vi "Limit Test.vi"(7 "CallingVI":refnum<vi>, 8 "error in":errorcluster, 9 "Previous":dbl, 10 "Setpoint in":dbl, 11 "Limits in":cluster{"Maximum":dbl, "Minimum":dbl}) -> (0 "error out":errorcluster, 2 "Setpoint out":dbl, 3 "Limits out":cluster{"Maximum":dbl, "Minimum":dbl})   [LabVIEW 2023, in "Instruments.lvlib" / "Instruments.lvclass"]
doc: "This routine tests limits provided by the caller routine and generates a warning if the value is out of range."
uses:
  Library/Instruments.lvclass
  <vilib>/ErrorRing/Error Ring.xnode
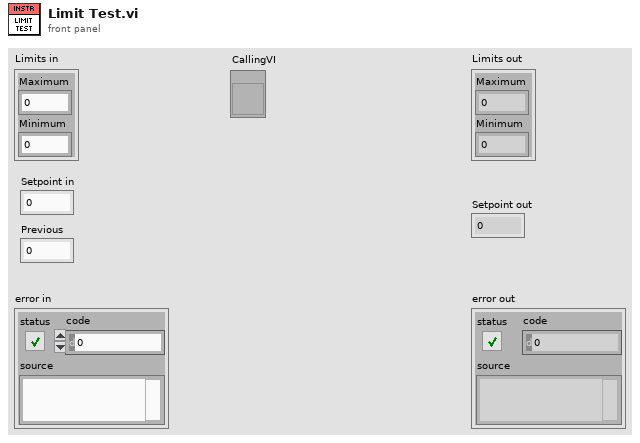
[diagram p1: front panel]
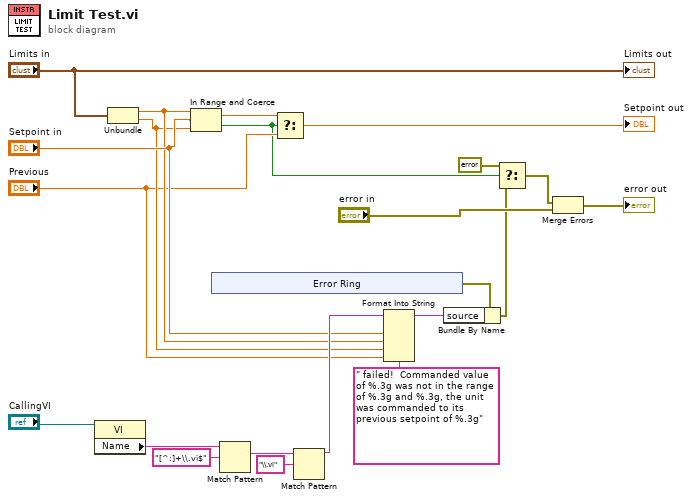
[diagram p0: block diagram]
diagram:
  n1 = property class="VI"(reference="CallingVI") -> ("Name"=w15:string)  [unwired: 1 in, 2 out]
  n2 = Unbundle("Limits in") -> ("Maximum"=w11:dbl, "Minimum"=w10:dbl)
  n3 = In Range and Coerce(upper limit=w11, x="Setpoint in", lower limit=w10) -> (coerced(x)=w21:dbl, In Range?=w6:bool)
  n4 = xnode "Error Ring"() -> ("error out"=w8:errorcluster)
  n5 = Match Pattern(string=w15, regular expression="[^:]+\\.vi$") -> (match substring=w17:string)  [unwired: 1 in, 3 out]
  n6 = Select(t=w21, s=w6, f="Previous") -> (s? t:f=→"Setpoint out":dbl)
  n7 = Match Pattern(string=w17, regular expression="\\.vi") -> (before substring=w13:string)  [unwired: 1 in, 3 out]
  n8 = Format Into String(format string=" failed!  Commanded value of %.3g was not in the range of %.3g and %.3g, the unit was commanded to its previous setpoint of %.3g", initial string=w13, "Setpoint in", w11, w10, "Previous") -> (resulting string=w7:string)  [unwired: 1 in, 1 out]
  n9 = Bundle By Name(cluster=w8, "source"=w7) -> (w2:errorcluster)
  n10 = Select(t=errorcluster {"status"=FALSE, "code"=0, "source"=""}, s=w6, f=w2) -> (s? t:f=w5:errorcluster)
  n11 = Merge Errors(w5, "error in") -> (→"error out":errorcluster)
  "Limits out" <- "Limits in"
